vi "Search for Attribute by Type.vi"(5 "Recurse Up List":bool, 6 "Names":string[](array[string]), 7 "Linked List ID":string, 8 "error in (no error)":errorcluster, 9 "Attributes":variant[](array[variant]), 10 "IDs":string[](array[string]), 11 "Linked List in":refnum<class "Linked List.lvclass">) -> (0 "error out":errorcluster, 1 "Attributes":variant[](array[variant]), 2 "IDs":string[](array[string]), 3 "Linked List out":refnum<class "Linked List.lvclass">, 4 "Names":string[](array[string]))   [LabVIEW 2019, in "Linked Lists.lvlib" / "Linked List.lvclass"]
uses:
  <vilib>/gpm_packages/@cs/linked-list/Source/Linked List/Linked List/Linked List.lvclass
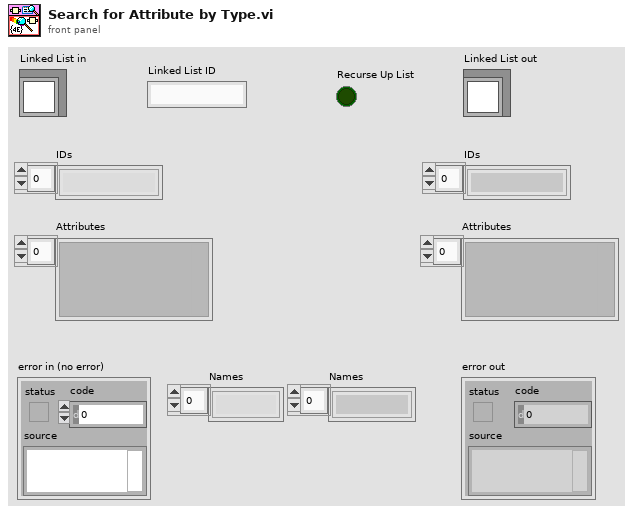
[diagram p1: front panel]
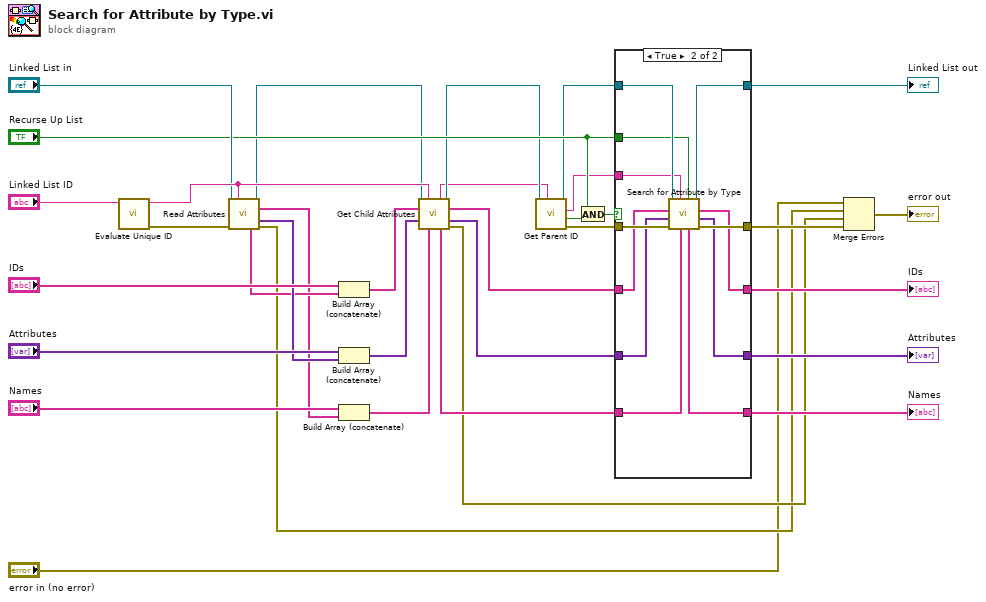
[diagram p0: block diagram]
diagram:
  n1 = call <vilib>:"Evaluate Unique ID.vi"("Unique ID"="Linked List ID") -> ("error out"=w33:errorcluster, "Unique ID Out"=w32:string)  [unwired: 9 in]
  n2 = call-dynamic "Read Attributes.vi"("Linked List in"="Linked List in", "Linked List ID"=w32, "error in (no error)"=w33) -> ("Linked List out"=w13:refnum<class "Linked List.lvclass">, "Attribute Names out"=w15:string[], "Attributes"=w21:variant[], "Data IDs"=w16:string[], "error out"=w2:errorcluster)  [unwired: 6 in, 2 out]
  n3 = Build Array (concatenate)("IDs", w16) -> (w6:string[])
  n4 = Build Array (concatenate)("Attributes", w21) -> (w8:variant[])
  n5 = Build Array (concatenate)("Names", w15) -> (w10:string[])
  n6 = call <vilib>:"Get Child Attributes.vi"("Linked List in"=w13, "Linked List ID"=w32, "IDs"=w6, "Attributes"=w8, "Names"=w10) -> ("Linked List ID out"=w11:string, "Linked List out"=w12:refnum<class "Linked List.lvclass">, "IDs"=w5:string[], "Attributes"=w7:variant[], "Names"=w9:string[], "error out"=w3:errorcluster)  [unwired: 4 in, 1 out]
  n7 = call-dynamic "Get Parent ID.vi"("Linked List ID"=w11, "Linked List in"=w12) -> ("error out"=w19:errorcluster, "Valid Parent ID"=w18:bool, "Parent ID"=w17:string, "Linked List out"=w20:refnum<class "Linked List.lvclass">)  [unwired: 6 in]
  n8 = And(x="Recurse Up List", y=w18) -> (x .and. y?=w14:bool)
  n9 = case shown="True" w14 {
    tunnel: [w38 w51] -> w29
    tunnel: w19 -> [w38 w50]
    tunnel: w20 -> [w39 w49]
    tunnel: [w39 w48] -> w30
    tunnel: [w37 w47] -> w28
    tunnel: w5 -> [w37 w46]
    tunnel: w17 -> [_ w45]
    tunnel: w7 -> [w36 w44]
    tunnel: [w36 w43] -> w25
    tunnel: w9 -> [w35 w42]
    tunnel: [w35 w41] -> w23
    tunnel: "Recurse Up List" -> [_ w40]
    frame False {
    }
    frame True {
      n10 = call-dynamic "Search for Attribute by Type.vi"("Recurse Up List"=w40, "Names"=w42, "Linked List ID"=w45, "error in (no error)"=w50, "Attributes"=w44, "IDs"=w46, "Linked List in"=w49) -> ("error out"=w51:errorcluster, "Attributes"=w43:variant[], "IDs"=w47:string[], "Linked List out"=w48:refnum<class "Linked List.lvclass">, "Names"=w41:string[])
    }
  }
  "Linked List out" <- w30
  "IDs" <- w28
  "Attributes" <- w25
  "Names" <- w23
  n11 = Merge Errors("error in (no error)", w2, w3, w29) -> (→"error out":errorcluster)
